vi "New Topic.vi"(9 "Data Type":variant, 10 "Name":string) -> (0 "error out":errorcluster, 3 "Topic out":refnum<class "Topic.lvclass">)   [LabVIEW 2015, in "Mediator.lvlib" / "Topic.lvclass"]
uses:
  Topic.lvclass
  Topic.lvclass/Topic.ctl
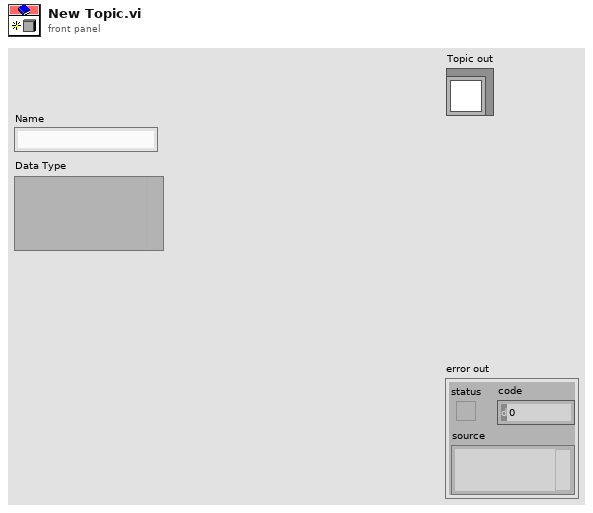
[diagram p1: front panel]
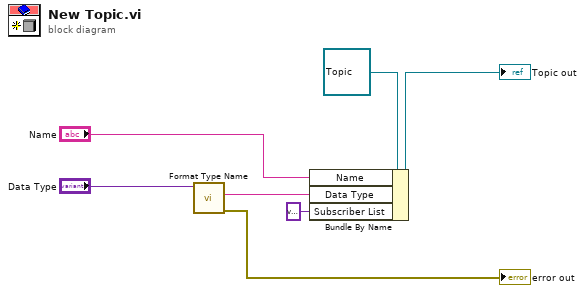
[diagram p0: block diagram]
diagram:
  n1 = call "Format Type Name.vi"("Data Type"="Data Type") -> ("error out"=→"error out":errorcluster, "Name"=w3:string)  [unwired: 9 in]
  n2 = Bundle By Name(cluster=refnum<class "Topic.lvclass"> refnum ("Topic in"), "Name"="Name", "Data Type"=w3, "Subscriber List"=variant) -> (→"Topic out":refnum<class "Topic.lvclass">)
